vi "MKS CTLR - Master.vi"() -> (2 "Baratron\n(Torr)":dbl, 3 "Separator Flow\n(SCCM)":dbl, 4 "Target Cavity Flow\n(SCCM)":dbl, 5 "MKS946 High Pressure\n(Torr)":dbl)   [LabVIEW 2013]
panel:
  in  "MKS 946 Vacuum Systerm\n VISA resource in":refnum<visa-resource-name>
  in  "MKS 670 High Accuracy\nSignal Conditioner\nVISA rresource in":refnum<visa-resource-name>
  in  "MKS 670 Error In":errorcluster
  in  "MKS 946 Error In":errorcluster
  out "MKS 946 Error Out":errorcluster
  out "Target String":string
  out "Separator String":string
  out "High Pressure String":string
  out "MKS 670 Error Out":errorcluster
  out "Baratron String":string
  out "Measurements":i32
  in  "stop":bool
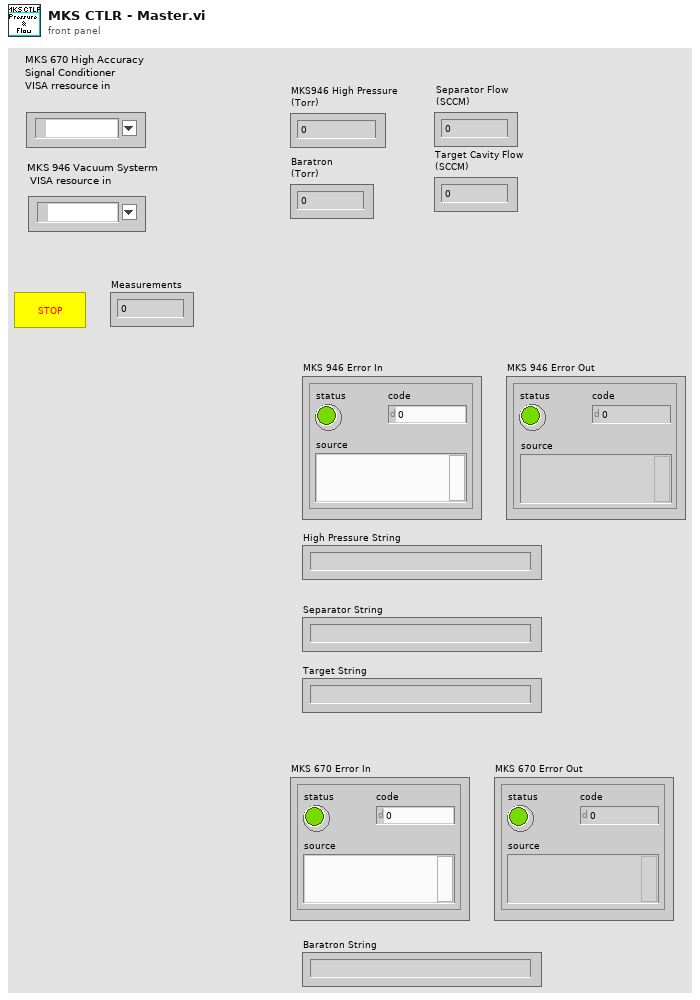
[diagram p1: front panel]
types:
  T1 = enum16{"MKS946 High Pressure Gauge", "MKS946 Separator Flow", "MKS946 Target Cavity Flow", "MKS670 Low Pressure Gauge"}
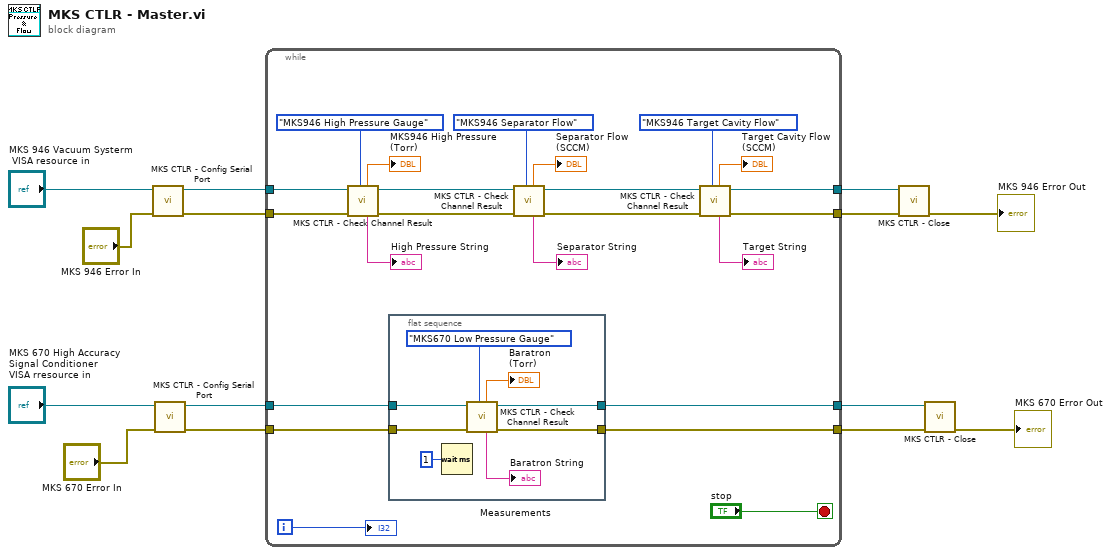
[diagram p0: block diagram]
diagram:
  n1 = call "MKS CTLR - Config Serial Port.vi"("Error In"="MKS 946 Error In", "MKS ViiSA resource name in"="MKS 946 Vacuum Systerm\n VISA resource in") -> ("Error Out"=w8:errorcluster, "VISA resource name out"=w9:refnum<visa-resource-name>)  [unwired: 8 in]
  n2 = call "MKS CTLR - Config Serial Port.vi"("Error In"="MKS 670 Error In", "MKS ViiSA resource name in"="MKS 670 High Accuracy\nSignal Conditioner\nVISA rresource in") -> ("Error Out"=w13:errorcluster, "VISA resource name out"=w14:refnum<visa-resource-name>)  [unwired: 8 in]
  n3 = while {
    tunnel: w14 -> [w35]
    tunnel: w13 -> [w34]
    tunnel: [w33] -> w10
    tunnel: [w32] -> w11
    tunnel: w8 -> [w29]
    tunnel: w9 -> [w28]
    tunnel: [w17] -> w6
    tunnel: [w16] -> w5
    i -> [w36]
    stop <- "stop" stop-if-true
    n4 = call "MKS CTLR - Check Channel Result.vi"("Channel"=T1."MKS946 High Pressure Gauge", "error in (no error)"=w29, "VISA resource name (IN)"=w28) -> ("error out"=w23:errorcluster, "VISA resource name (OUT)"=w24:refnum<visa-resource-name>, "String Value"=→"High Pressure String":string, "Pressure value"=→"MKS946 High Pressure\n(Torr)":dbl)  [unwired: 5 in]
    n5 = flat-sequence {
      tunnel: w35 -> [w43]
      tunnel: w34 -> [w42]
      tunnel: [w41] -> w33
      tunnel: [w40] -> w32
      frame #0 {
        n6 = Wait (ms)(milliseconds to wait=u32 1) -> ()  [unwired: 1 out]
        n7 = call "MKS CTLR - Check Channel Result.vi"("Channel"=T1."MKS670 Low Pressure Gauge", "error in (no error)"=w42, "VISA resource name (IN)"=w43) -> ("error out"=w41:errorcluster, "VISA resource name (OUT)"=w40:refnum<visa-resource-name>, "String Value"=→"Baratron String":string, "Pressure value"=→"Baratron\n(Torr)":dbl)  [unwired: 5 in]
      }
    }
    n8 = call "MKS CTLR - Check Channel Result.vi"("Channel"=T1."MKS946 Separator Flow", "error in (no error)"=w23, "VISA resource name (IN)"=w24) -> ("error out"=w18:errorcluster, "VISA resource name (OUT)"=w19:refnum<visa-resource-name>, "String Value"=→"Separator String":string, "Pressure value"=→"Separator Flow\n(SCCM)":dbl)  [unwired: 5 in]
    n9 = call "MKS CTLR - Check Channel Result.vi"("Channel"=T1."MKS946 Target Cavity Flow", "error in (no error)"=w18, "VISA resource name (IN)"=w19) -> ("error out"=w16:errorcluster, "VISA resource name (OUT)"=w17:refnum<visa-resource-name>, "String Value"=→"Target String":string, "Pressure value"=→"Target Cavity Flow\n(SCCM)":dbl)  [unwired: 5 in]
    "Measurements" <- w36
  }
  n10 = call "MKS CTLR - Close.vi"("error in (no error)"=w5, "VISA resource name (IN)"=w6) -> ("error out"=→"MKS 946 Error Out":errorcluster)  [unwired: 9 in]
  n11 = call "MKS CTLR - Close.vi"("error in (no error)"=w10, "VISA resource name (IN)"=w11) -> ("error out"=→"MKS 670 Error Out":errorcluster)  [unwired: 9 in]
